vi "Picture Size Read.vi"(4 "error in (no error)":errorcluster, 6 "Container State":T4, 7 "Display State In":T2={"Persistent"={"Elements"=[], "PicElements"=[], "Limits"=[], "Selection"=[], "Selection Color"=0, "Highlight"=[], "Highlight Val"=0, "Highlight Color"={"Back"=0, "Edge"=0}, "Font"={"Details"={"Font Name:"="Lucida Sans", "Size"=24, "Strikeout?"=FALSE, "Italic?"=FALSE, "Underline?"=FALSE, "Outline?"=FALSE, "Shadow?"=FALSE, "Bold?"=TRUE}, "Color"=7697781}, "Bakground Color"=0}, "List Ref"=refnum, "nbVisible"=0, "FirstIdx"=0, "More.Width"=0}) -> (0 "error out":errorcluster, 2 "Value":T1, 3 "Display State Out":T2={"Persistent"={"Elements"=[], "PicElements"=[], "Limits"=[], "Selection"=[], "Selection Color"=0, "Highlight"=[], "Highlight Val"=0, "Highlight Color"={"Back"=0, "Edge"=0}, "Font"={"Details"={"Font Name:"="Lucida Sans", "Size"=24, "Strikeout?"=FALSE, "Italic?"=FALSE, "Underline?"=FALSE, "Outline?"=FALSE, "Shadow?"=FALSE, "Bold?"=TRUE}, "Color"=7697781}, "Bakground Color"=0}, "List Ref"=refnum, "nbVisible"=0, "FirstIdx"=0, "More.Width"=0})   [LabVIEW 2016, in "Horizontal MenuList.xctl"]
uses:
  Horizontal MenuList.xctl
  <vilib>/_xctls/Container State.ctl
  Horizontal MenuList_State.ctl
  _SubVIs/Highlight Colors.ctl
  <vilib>/Utility/miscctls.llb/LVBoundsTypeDef.ctl
  <vilib>/_xctls/XControlSupport.lvlib
panel:
  # "Replace the Value Indicator below with an Indicator of desired type.\nDo not remove this Indicator or the others from the connector pane. \nDo not change the connector pane pattern.\nThe Value Indicator should always be the second terminal from top on the output side in the connector pane."
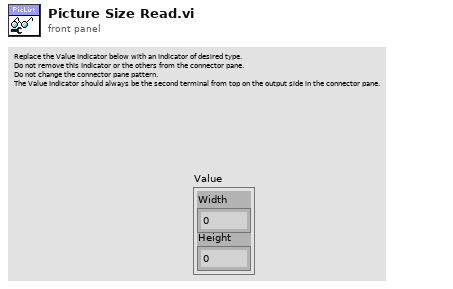
[diagram p1: front panel]
types:
  T1 = typedef "LVBoundsTypeDef.ctl" = cluster{"Width":u32, "Height":u32}
  T2 = typedef "Horizontal MenuList.xctl/Horizontal MenuList_State.ctl" = cluster{"Persistent":cluster{"Elements":string[], "PicElements":picture[], "Limits":i32[], "Selection":picture[], "Selection Color":u32, "Highlight":picture[], "Highlight Val":i32, "Highlight Color":T3, "Font":cluster{"Details":cluster{"Font Name:":string, "Size":i16, "Strikeout?":bool, "Italic?":bool, "Underline?":bool, "Outline?":bool, "Shadow?":bool, "Bold?":bool}, "Color":u32}, "Bakground Color":u32}, "List Ref":refnum<vi>, "nbVisible":u8, "FirstIdx":u8, "More.Width":u8}
  T3 = typedef "Horizontal MenuList.xctl/Highlight Colors.ctl" = cluster{"Back":u32, "Edge":u32}
  T4 = typedef "XControlSupport.lvlib/Container State.ctl" = cluster{"Indicator?":bool, "Run Mode?":bool, " Refnum":refnum<vi>}
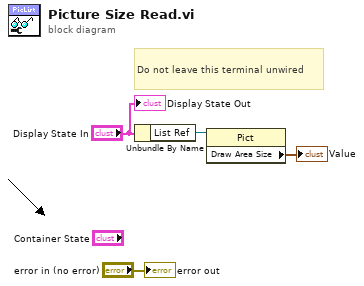
[diagram p0: block diagram]
diagram:
  # "Do not leave this terminal unwired"
  n1 = Unbundle By Name("Display State In") -> ("List Ref"=w2:refnum<vi>)
  n2 = property class="Pict"(reference=w2) -> ("Draw Area Size"=→"Value":T1)  [unwired: 1 in, 2 out]
  "error out" <- "error in (no error)"
  "Display State Out" <- "Display State In"
